vi "set_params.vi"(8 "error in (no error)":errorcluster caption="entrée d'erreur (pas d'erreur)", 11 "PassiveAggressiveClassifier.lvclass 2":refnum<class "PassiveAggressiveClassifier.lvclass">) -> (0 "error out":errorcluster caption="sortie d'erreur", 3 "PassiveAggressiveClassifier.lvclass":refnum<class "PassiveAggressiveClassifier.lvclass">)   [LabVIEW 2020, in "PassiveAggressiveClassifier.lvclass"]
uses:
  PassiveAggressiveClassifier.lvclass
  PassiveAggressiveClassifier.lvclass/PassiveAggressiveClassifier.ctl
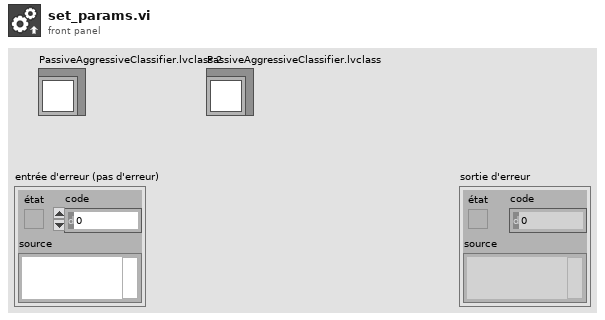
[diagram p1: front panel]
types:
  T1 = typedef "passive_aggressive_classifier_params.ctl" = cluster{"C":dbl, "fit_intercept":bool, "max_iter":dbl, "tol":cluster{"tol_type":string, "tol_float":dbl}, "early_stopping":bool, "validation_fraction":dbl, "n_iter_no_change":dbl, "shuffle":bool, "verbose":dbl, "loss":string, "n_jobs":dbl, "random_state":dbl, "warm_start":bool, "class_weight":cluster{"class_weight_type":string, "class_weight_dict":string}, "average":bool}
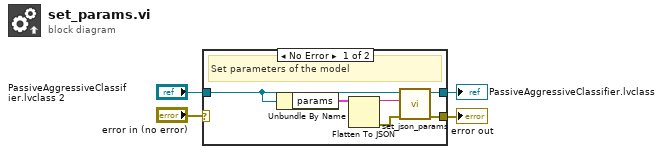
[diagram p0: block diagram]
diagram:
  n1 = case shown="No Error" "error in (no error)" {
    selector: "error in (no error)" -> [_ w12]
    tunnel: [w7 w12] -> w3
    tunnel: [w8 w11] -> w1
    tunnel: "PassiveAggressiveClassifier.lvclass 2" -> [w5 w11]
    frame No Error {
      # "Set parameters of the model"
      n2 = Unbundle By Name(w5) -> ("params"=w10:T1)
      n3 = Flatten To JSON(anything=w10) -> (JSON string=w9:string, 11:w6:errorcluster)  [unwired: 2 in]
      n4 = call-dynamic "set_json_params.vi"("error in (no error)"=w6, "params"=w9, "Model en entrée"=w5) -> ("error out"=w7:errorcluster, "Model en sortie"=w8:refnum<class "PassiveAggressiveClassifier.lvclass">)  [unwired: 7 in]
    }
    frame Error {
    }
  }
  "error out" <- w3
  "PassiveAggressiveClassifier.lvclass" <- w1
